vi "TestExec.Configure Setup and Dialog - Station.vi"(9 "Dialog":bool, 10 "SectAddFiles":string[](array[string])=["AdditionalConfig"] caption="Sections with Additional Files", 11 "Local Station Folder":path=path "C:/MTE/Test Executive/Config") -> (1 "Saved":bool, 2 "Data Out":variant, 3 "AppData out":refnum<class "Class.AppData.lvclass">)   [LabVIEW 2018]
uses:
  Common/Utils/TestExec/TestExec.WorkingDir.ctl
  <vilib>/KATE/Config/App Data/Class.AppData.lvclass
  Controls and Type Defs/TestExec.Config Dialog State.ctl
  <vilib>/Utility/config.llb/Write Key (String).vi
  <vilib>/KATE/Files/File Utils.lvlib
  <vilib>/Utility/config.llb/NI_LVConfig.lvlib
panel:
  out "Tab Control":enum32{"Inputs", "Data", "Outputs"}(tab)
  in  "Open Local Station File on Save":bool
  out "Exists_CfgFiles":bool[](array[boolean])
  out "Exists_ModeCfg":bool
  in  "Sequence":cluster{"Default":string}={"Default"="Undefined"}
  in  "Factory":cluster{"Location":string}={"Location"="Undefined"}
  in  "Route Check Enable":bool
  in  "Facility":cluster{"Name":string, "Location":string}={"Name"="Undefined", "Location"="Undefined"}
  in  "Station":T1={"Name"="Undefined", "PN"="Undefined", "SN"="Undefined", "Rev"="Undefined"}
  out "Additional Config Files":path[](array[path])
  in  "Mode Config File":path
  out "Local Station Config File":path=path "C:/MTE/Data/Eyetube Calibration/Capture"
  in  "Save":bool
  in  "Cancel":bool
  in  "Data Folders":T2[](array[typedef])=[{"Name"="ResultsLocalDir", "Path"=path "c:/MTE/Data/XML"}, {"Name"="ResultsExternalDir", "Path"=path "c:/MTE/Data/Results"}, {"Name"="DataArchiveDir", "Path"=path "c:/MTE/Data/Archive"}, {"Name"="DataSumArchiveDir", "Path"=path "c:/MTE/Data/ArchiveSum"}]
  # "Test Station Configuration"
  # "Name                                                                                                         Path"
  # "If this is empty, the default modes will be used."
  # "If a file is specified, it's contents will over write local settings."
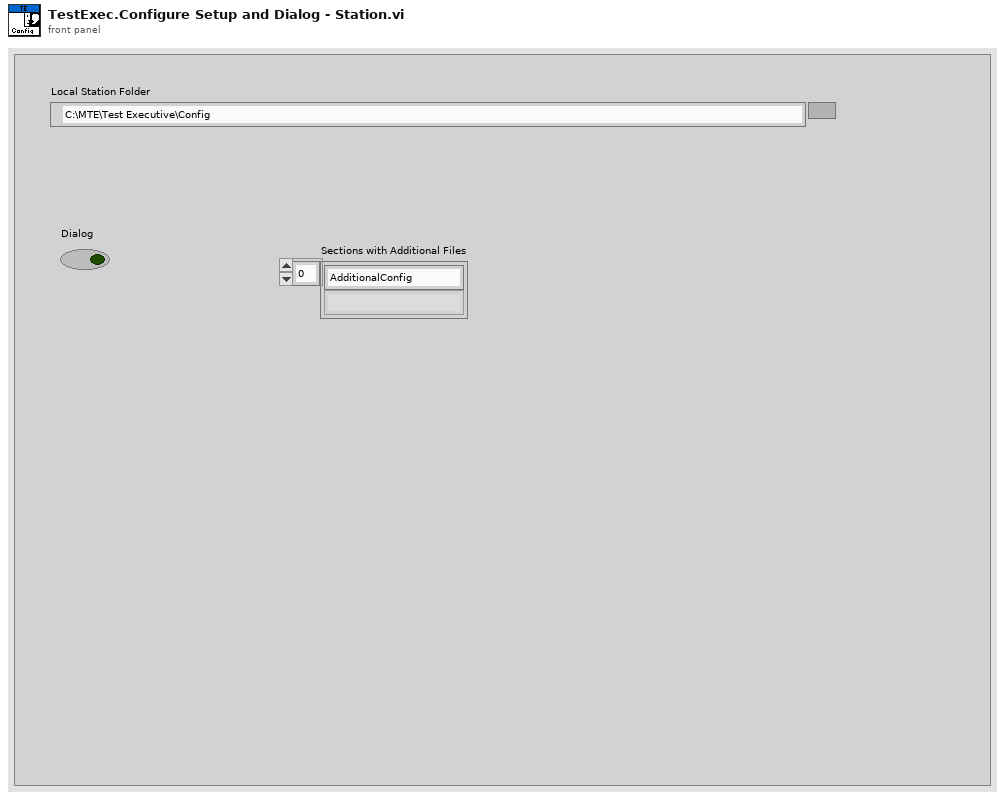
[diagram p1: front panel]
types:
  T1 = cluster{"Name":string, "PN":string, "SN":string, "Rev":string}
  T2 = typedef "TestExec.WorkingDir.ctl" = cluster{"Name":string, "Path":path}
  T3 = typedef "TestExec.Config Dialog State.ctl" = enum16{"Init", "Set Defaults", "Load Config", "Initialize Config", "Initialize Output", "Dialog", "Save", "Update Output", "Done"}
  T4 = enum32{"Invalid", "Standard", "Closed", "Hidden", "Minimized", "Maximized"}
  T5 = cluster{"Local Station Folder":path, "LocalCfgFile":path, "State":T3, "Save":bool, "Config":refnum<class "Class.AppData.lvclass">}
  T6 = typedef "NI_LVConfig.lvlib/Config Data RefNum.ctl" = refnum<k1>
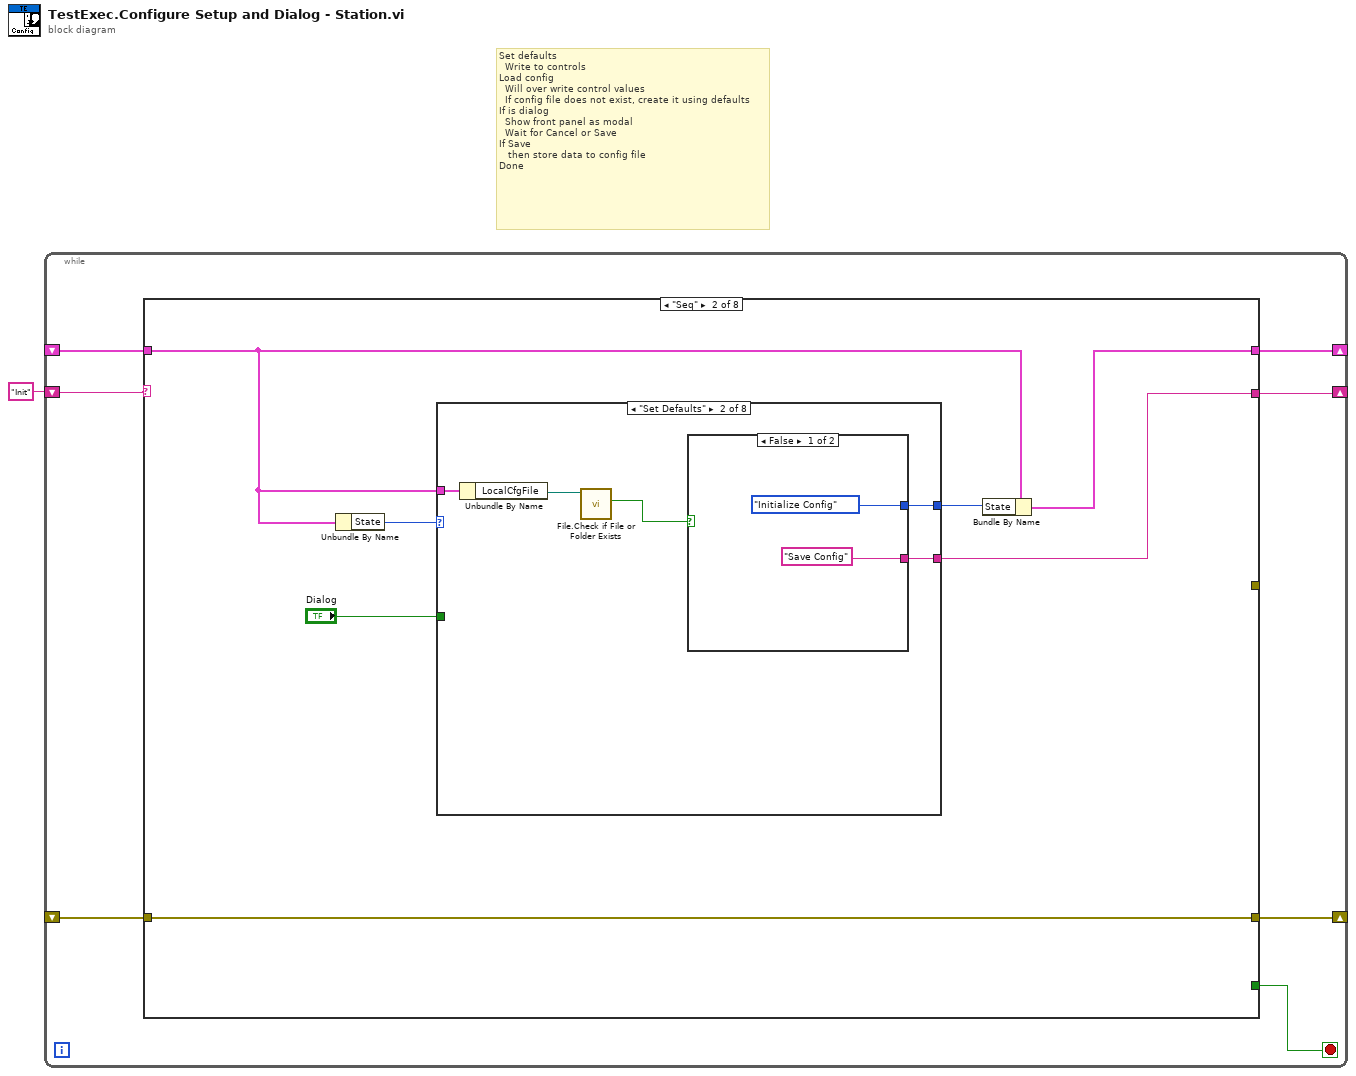
[diagram p0: block diagram]
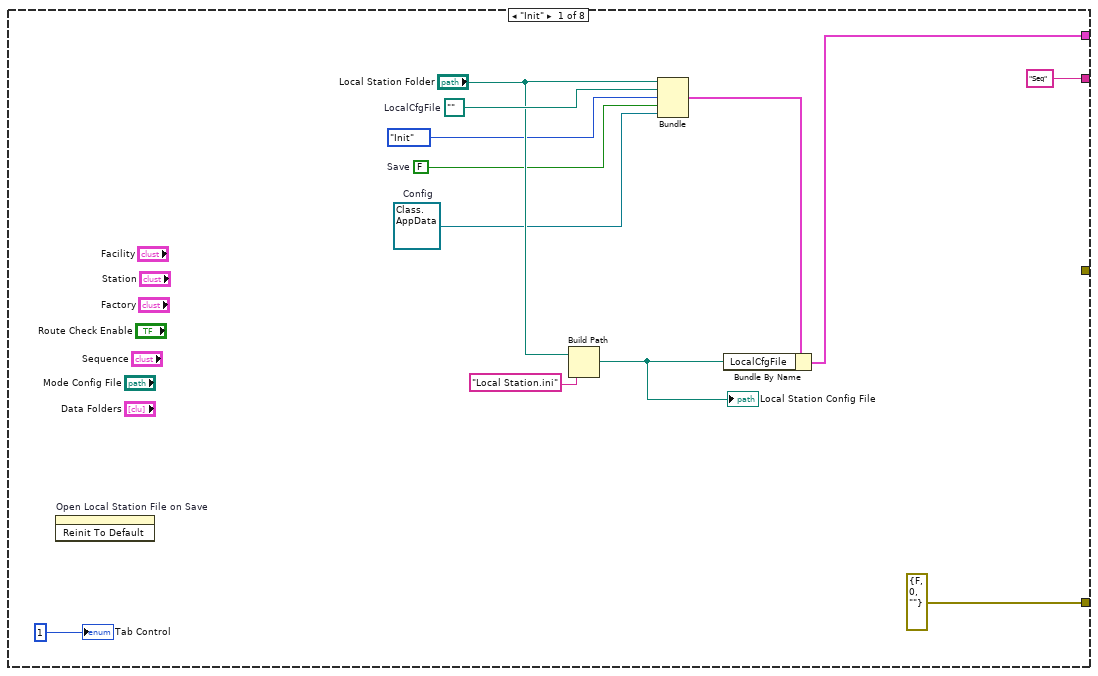
[diagram p2: hidden frame]
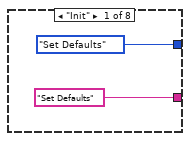
[diagram p3: hidden frame]
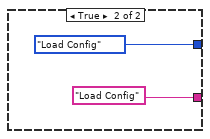
[diagram p4: hidden frame]
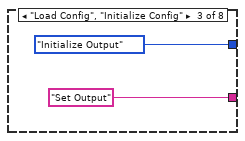
[diagram p5: hidden frame]
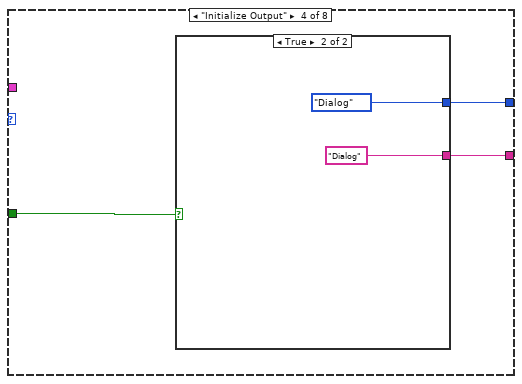
[diagram p6: hidden frame]
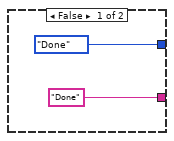
[diagram p7: hidden frame]
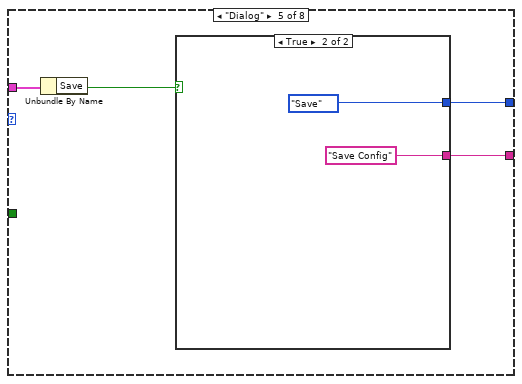
[diagram p8: hidden frame]
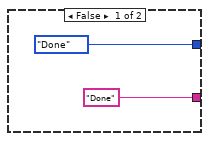
[diagram p9: hidden frame]
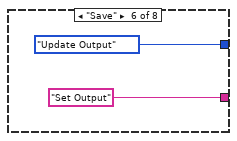
[diagram p10: hidden frame]
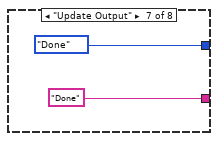
[diagram p11: hidden frame]
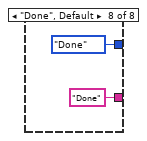
[diagram p12: hidden frame]
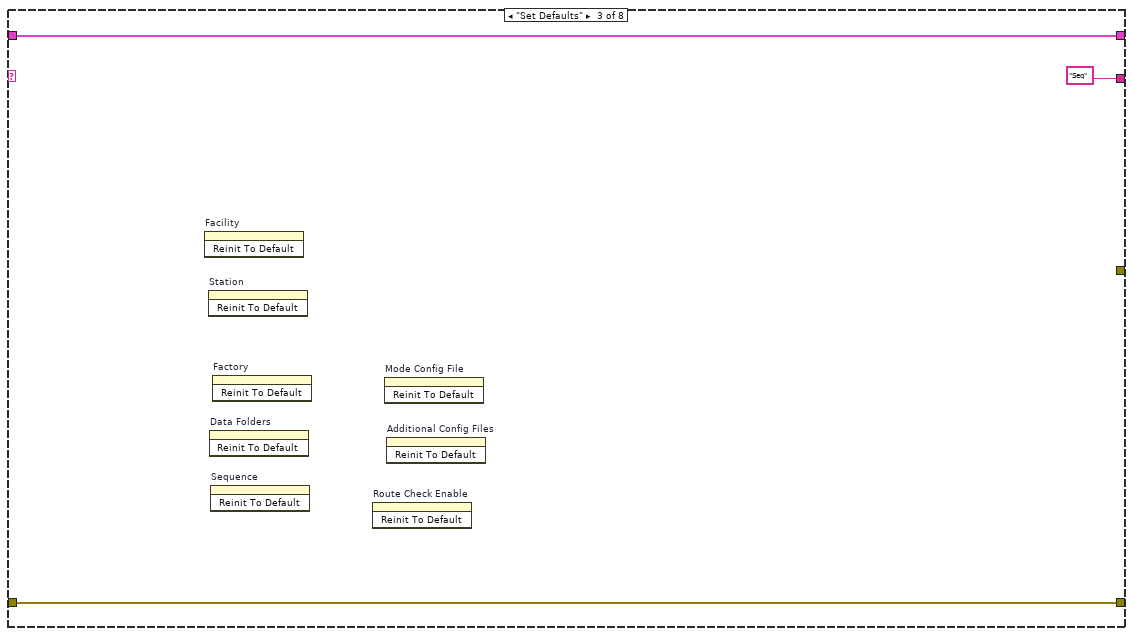
[diagram p13: hidden frame]
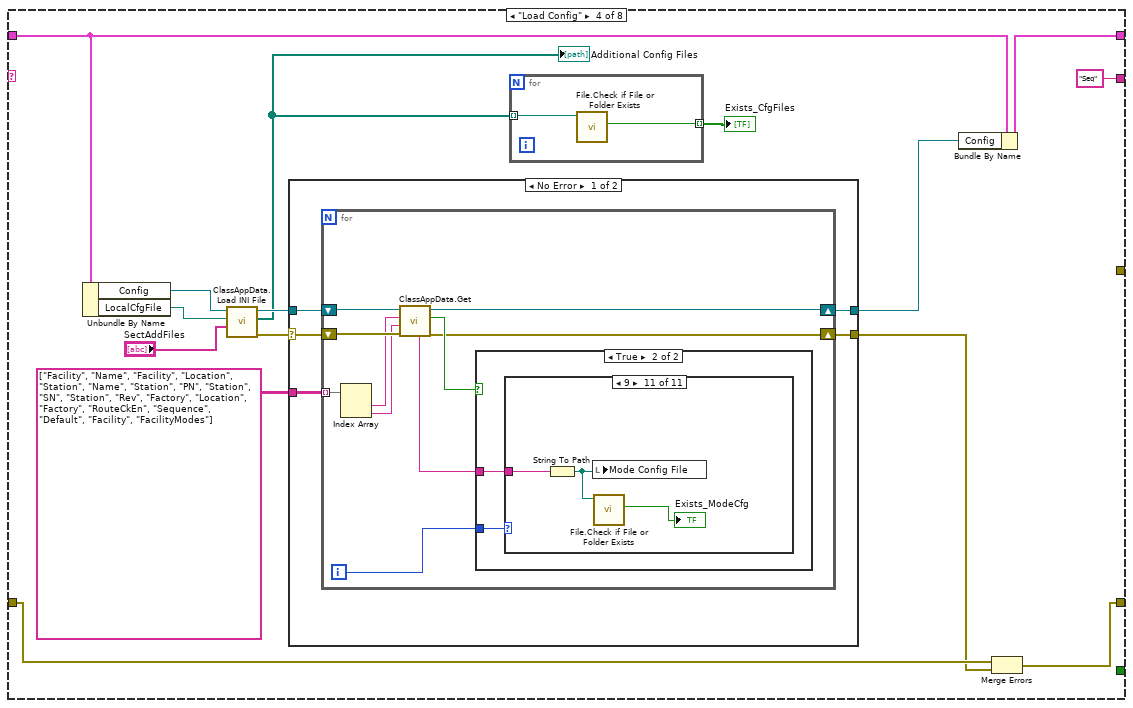
[diagram p14: hidden frame]
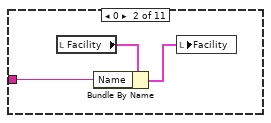
[diagram p17: hidden frame]
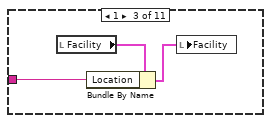
[diagram p18: hidden frame]
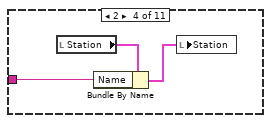
[diagram p19: hidden frame]
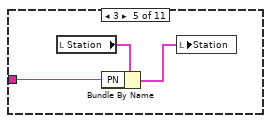
[diagram p20: hidden frame]
diagram:
  # "Set defaults\n  Write to controls\nLoad config\n  Will over write control values\n  If config file does not exist, create it using defaults\nIf is dialog\n  Show front panel as modal\n  Wait for Cancel or Save\nIf Save\n   then store data to config file\nDone"
  n1 = while {
    shift-right: [w6] -> _
    shift-left: _ -> [w8]
    shift-right: [w4] -> _
    shift-left: "Init" -> [w7]
    shift-right: [w2] -> _
    shift-left: _ -> [w3]
    stop <- w5 stop-if-true
    n2 = case shown="\"Seq\"" w7 {
      tunnel: w8 -> [_ w25 w63 w78 w150 w190 w200 w217]
      tunnel: [w15 w24 w63 w77 w149 w190 w199 w217] -> w6
      tunnel: ["Seq" w22 "Seq" "Seq" "Seq" "Seq" w198 "Done"] -> w4
      tunnel: [_ _ _ _ _ _ _ TRUE] -> w5
      tunnel: [_ _ _ _ w140 _ _ _] -> _
      tunnel: w3 -> [_ w21 w62 w68 w139 w196 w197 w218]
      tunnel: [errorcluster {"status"=FALSE, "code"=0, "source"=""} ("error constant") w21 w62 w66 w136 w196 w197 w218] -> w2
      frame "Init" {
        w10 = refnum<class "Class.AppData.lvclass"> refnum  # Config
        w13 = FALSE  # Save
        w18 = path ""  # LocalCfgFile
        n3 = invoke on="Open Local Station File on Save" class="Bool (strict)" method="Reinit To Default"() -> ()  [unwired: 3 in, 3 out]
        n4 = Build Path(base path="Local Station Folder", name or relative path="Local Station.ini") -> (appended path=w11:path)
        "Local Station Config File" <- w11
        n5 = Bundle("Local Station Folder"="Local Station Folder", "LocalCfgFile"=w18, "State"=TestExec.Config_Dialog_State."Init", "Save"=w13, "Config"=w10) -> (w16:T5)  [unwired: 1 in]
        n6 = Bundle By Name(cluster=w16, "LocalCfgFile"=w11) -> (w15:T5)
        "Tab Control" <- 1
      }
      frame "Seq" {
        n7 = Unbundle By Name(w25) -> ("State"=w27:T3)
        n8 = case shown="\"Set Defaults\"" w27 {
          tunnel: "Dialog" -> [_ _ _ w43 _ _ _ _]
          tunnel: w25 -> [_ w34 _ _ w49 _ _ _]
          tunnel: [TestExec.Config_Dialog_State."Set Defaults" ("State") w31 TestExec.Config_Dialog_State."Initialize Output" ("State") w42 w51 TestExec.Config_Dialog_State."Update Output" ("State") TestExec.Config_Dialog_State."Done" ("State") TestExec.Config_Dialog_State."Done" ("State")] -> w23
          tunnel: ["Set Defaults" w30 "Set Output" w41 w50 "Set Output" "Done" "Done"] -> w22
          frame "Init" {
          }
          frame "Set Defaults" {
            n9 = Unbundle By Name(w34) -> ("LocalCfgFile"=w33:path)
            n10 = call <vilib>:"File.Check if File or Folder Exists.vi"("Path"=w33) -> ("Exists"=w32:bool)  [unwired: 6 in, 4 out]
            n11 = case shown="False" w32 {
              tunnel: [TestExec.Config_Dialog_State."Initialize Config" ("State") TestExec.Config_Dialog_State."Load Config" ("State")] -> w31
              tunnel: ["Save Config" "Load Config"] -> w30
              frame False {
              }
              frame True {
              }
            }
          }
          frame "Load Config", "Initialize Config" {
          }
          frame "Initialize Output" {
            n12 = case shown="True" w43 {
              tunnel: [TestExec.Config_Dialog_State."Done" ("State") TestExec.Config_Dialog_State."Dialog" ("State")] -> w42
              tunnel: ["Done" "Dialog"] -> w41
              frame False {
              }
              frame True {
              }
            }
          }
          frame "Dialog" {
            n13 = Unbundle By Name(w49) -> ("Save"=w48:bool)
            n14 = case shown="True" w48 {
              tunnel: [TestExec.Config_Dialog_State."Done" ("State") TestExec.Config_Dialog_State."Save" ("State")] -> w51
              tunnel: ["Done" "Save Config"] -> w50
              frame False {
              }
              frame True {
              }
            }
          }
          frame "Save" {
          }
          frame "Update Output" {
          }
          frame "Done", Default {
          }
        }
        n15 = Bundle By Name(cluster=w25, "State"=w23) -> (w24:T5)
      }
      frame "Set Defaults" {
        n16 = invoke on="Facility" class="Clust (strict)" method="Reinit To Default"() -> ()  [unwired: 3 in, 3 out]
        n17 = invoke on="Station" class="Clust (strict)" method="Reinit To Default"() -> ()  [unwired: 3 in, 3 out]
        n18 = invoke on="Data Folders" class="Arr (strict)" method="Reinit To Default"() -> ()  [unwired: 3 in, 3 out]
        n19 = invoke on="Sequence" class="Clust (strict)" method="Reinit To Default"() -> ()  [unwired: 3 in, 3 out]
        n20 = invoke on="Factory" class="Clust (strict)" method="Reinit To Default"() -> ()  [unwired: 3 in, 3 out]
        n21 = invoke on="Route Check Enable" class="Bool (strict)" method="Reinit To Default"() -> ()  [unwired: 3 in, 3 out]
        n22 = invoke on="Mode Config File" class="Path" method="Reinit To Default"() -> ()  [unwired: 3 in, 3 out]
        n23 = invoke on="Additional Config Files" class="Arr (strict)" method="Reinit To Default"() -> ()  [unwired: 3 in, 3 out]
      }
      frame "Load Config" {
        n24 = Unbundle By Name(w78) -> ("Config"=w76:refnum<class "Class.AppData.lvclass">, "LocalCfgFile"=w75:path)
        n25 = call <vilib>:"ClassAppData.Load INI File.vi"("Sections that List RemoteFile"="SectAddFiles", "INI File"=w75, "Class - App Data in"=w76) -> ("error out"=w73:errorcluster, "Additional Cfg Files"=w69:path[], "Class - App Data out"=w74:refnum<class "Class.AppData.lvclass">)  [unwired: 6 in]
        "Additional Config Files" <- w69
        n26 = case shown="No Error" w73 {
          selector: w73 -> [w85 _]
          tunnel: w74 -> [w86 w133]
          tunnel: [w84 w133] -> w72
          tunnel: string[][] [["Facility", "Name"], ["Facility", "Location"], ["Station", "Name"], ["Station", "PN"], ["Station", "SN"], ["Station", "Rev"], ["Factory", "Location"], ["Factory", "RouteCkEn"], ["Sequence", "Default"], ["Facility", "FacilityModes"]] -> [w83 _]
          tunnel: [w82 _] -> w67
          frame No Error {
            n27 = for {
              shift-right: [w90] -> w84
              shift-left: w86 -> [w96]
              shift-right: [w89] -> w82
              shift-left: w85 -> [w95]
              tunnel: w83 -> [w94] mode=indexing
              i -> [w87]
              n28 = Index Array(array=w94) -> (element #1=w93:string, element #2=w92:string)  [unwired: 2 in]
              n29 = call <vilib>:"ClassAppData.Get.vi"("error in (no error)"=w95, "Name"=w92, "Section"=w93, "Class - App Data in"=w96) -> ("error out"=w89:errorcluster, "Found"=w91:bool, "Class - App Data out"=w90:refnum<class "Class.AppData.lvclass">, "String Data"=w88:string)  [unwired: 3 in, 1 out]
              n30 = case shown="True" w91 {
                tunnel: w88 -> [_ w97]
                tunnel: w87 -> [_ w98]
                frame False {
                  # "Skip"
                }
                frame True {
                  n31 = case shown="9" w98 {
                    tunnel: w97 -> [_ w99 w102 w105 w108 w111 w114 w117 w125 w127 w132]
                    frame Default {
                    }
                    frame 0 {
                      n32 = local read "Facility"() -> (w101:cluster{"Name":string, "Location":string})
                      n33 = Bundle By Name(cluster=w101, "Name"=w99) -> (w100:cluster{"Name":string, "Location":string})
                      n34 = local write "Facility"(w100) -> ()
                    }
                    frame 1 {
                      n35 = local read "Facility"() -> (w104:cluster{"Name":string, "Location":string})
                      n36 = Bundle By Name(cluster=w104, "Location"=w102) -> (w103:cluster{"Name":string, "Location":string})
                      n37 = local write "Facility"(w103) -> ()
                    }
                    frame 2 {
                      n38 = local read "Station"() -> (w107:T1)
                      n39 = Bundle By Name(cluster=w107, "Name"=w105) -> (w106:T1)
                      n40 = local write "Station"(w106) -> ()
                    }
                    frame 3 {
                      n41 = local read "Station"() -> (w110:T1)
                      n42 = Bundle By Name(cluster=w110, "PN"=w108) -> (w109:T1)
                      n43 = local write "Station"(w109) -> ()
                    }
                    frame 4 {
                      n44 = local read "Station"() -> (w113:T1)
                      n45 = Bundle By Name(cluster=w113, "SN"=w111) -> (w112:T1)
                      n46 = local write "Station"(w112) -> ()
                    }
                    frame 5 {
                      n47 = local read "Station"() -> (w116:T1)
                      n48 = Bundle By Name(cluster=w116, "Rev"=w114) -> (w115:T1)
                      n49 = local write "Station"(w115) -> ()
                    }
                    frame 6 {
                      n50 = local read "Factory"() -> (w119:cluster{"Location":string})
                      n51 = Bundle By Name(cluster=w119, "Location"=w117) -> (w118:cluster{"Location":string})
                      n52 = local write "Factory"(w118) -> ()
                    }
                    frame 7 {
                      n53 = To Upper Case(1:w125) -> (0:w126:string)
                      n54 = Equal?(x="1" ("y"), y=w125) -> (x = y?=w121:bool)
                      n55 = Equal?(x=w126, y="TRUE") -> (x = y?=w122:bool)
                      n56 = Or(x=w121, y=w122) -> (x .or. y?=w120:bool)
                      n57 = local write "Route Check Enable"(w120) -> ()
                    }
                    frame 8 {
                      n58 = local read "Sequence"() -> (w129:cluster{"Default":string})
                      n59 = Bundle By Name(cluster=w129, "Default"=w127) -> (w128:cluster{"Default":string})
                      n60 = local write "Sequence"(w128) -> ()
                    }
                    frame 9 {
                      n61 = String To Path(string=w132) -> (path=w131:path)
                      n62 = local write "Mode Config File"(w131) -> ()
                      n63 = call <vilib>:"File.Check if File or Folder Exists.vi"("Path"=w131) -> ("Exists"=→"Exists_ModeCfg":bool)  [unwired: 6 in, 4 out]
                    }
                  }
                }
              }
            }
          }
          frame Error {
          }
        }
        n64 = for {
          tunnel: w69 -> [w81] mode=indexing
          tunnel: [w80] -> w70 mode=indexing
          n65 = call <vilib>:"File.Check if File or Folder Exists.vi"("Path"=w81) -> ("Exists"=w80:bool)  [unwired: 6 in, 4 out]
        }
        "Exists_CfgFiles" <- w70
        n66 = Bundle By Name(cluster=w78, "Config"=w72) -> (w77:T5)
        n67 = Merge Errors(w68, w67) -> (w66:errorcluster)
      }
      frame "Save Config" {
        n68 = Unbundle By Name(w150) -> ("LocalCfgFile"=w144:path, "Config"=w146:refnum<class "Class.AppData.lvclass">)
        n69 = call <vilib>:"Open Config Data.vi"("create file if necessary (T)"=TRUE, "configuration file path"=w144) -> ("error out"=w135:errorcluster, "refnum"=w143:T6)  [unwired: 7 in, 1 out]
        n70 = for {
          shift-right: [w162] -> w148
          shift-left: w146 -> [w165]
          shift-right: [w161] -> w138
          shift-left: errorcluster {"status"=FALSE, "code"=0, "source"=""} ("error constant") -> [w164]
          tunnel: string[][] [["Facility", "Name"], ["Facility", "Location"], ["Station", "Name"], ["Station", "PN"], ["Station", "SN"], ["Station", "Rev"], ["Factory", "Location"], ["Factory", "RouteCkEn"], ["Sequence", "Default"], ["Facility", "FacilityModes"]] -> [w163] mode=indexing
          shift-right: [w152] -> w137
          shift-left: w135 -> [w157]
          shift-right: [w153] -> w141
          shift-left: w143 -> [w158]
          i -> [w160]
          n71 = Index Array(array=w163) -> (element #1=w155:string, element #2=w156:string)  [unwired: 2 in]
          n72 = case shown="9" w160 {
            tunnel: [_ w166 w168 w171 w173 w175 w177 w179 w180 w184 w187] -> w154
            frame Default {
            }
            frame 0 {
              n73 = local read "Facility"() -> (w167:cluster{"Name":string, "Location":string})
              n74 = Unbundle By Name(w167) -> ("Name"=w166:string)
            }
            frame 1 {
              n75 = local read "Facility"() -> (w169:cluster{"Name":string, "Location":string})
              n76 = Unbundle By Name(w169) -> ("Location"=w168:string)
            }
            frame 2 {
              n77 = local read "Station"() -> (w170:T1)
              n78 = Unbundle By Name(w170) -> ("Name"=w171:string)
            }
            frame 3 {
              n79 = local read "Station"() -> (w172:T1)
              n80 = Unbundle By Name(w172) -> ("PN"=w173:string)
            }
            frame 4 {
              n81 = local read "Station"() -> (w174:T1)
              n82 = Unbundle By Name(w174) -> ("SN"=w175:string)
            }
            frame 5 {
              n83 = local read "Station"() -> (w176:T1)
              n84 = Unbundle By Name(w176) -> ("Rev"=w177:string)
            }
            frame 6 {
              n85 = local read "Factory"() -> (w178:cluster{"Location":string})
              n86 = Unbundle By Name(w178) -> ("Location"=w179:string)
            }
            frame 7 {
              n87 = local read "Route Check Enable"() -> (w181:bool)
              n88 = Select(t="TRUE" ("y"), s=w181, f="FALSE" ("y")) -> (s? t:f=w180:string)
            }
            frame 8 {
              n89 = local read "Sequence"() -> (w185:cluster{"Default":string})
              n90 = Unbundle By Name(w185) -> ("Default"=w184:string)
            }
            frame 9 {
              n91 = local read "Mode Config File"() -> (w188:path)
              n92 = call <vilib>:"File.Check if File or Folder Exists.vi"("Path"=w188) -> ("Exists"=w189:bool, "Dup Path"=w186:path)  [unwired: 6 in, 3 out]
              n93 = Path To String(path=w186) -> (string=w187:string)
              n94 = local write "Exists_ModeCfg"(w189) -> ()
            }
          }
          n95 = To Variant(anything=w154) -> (Variant=w159:variant)
          n96 = call <vilib>:"ClassAppData.Set.vi"("Section"=w155, "error in (no error)"=w164, "Value"=w159, "Name"=w156, "Class - App Data in"=w165) -> ("error out"=w161:errorcluster, "Class - App Data out"=w162:refnum<class "Class.AppData.lvclass">)  [unwired: 4 in, 1 out]
          n97 = call-poly <vilib>:"Write Key.vi"("section"=w155, "error in (no error)"=w157, "value"=w154, "key"=w156, "refnum"=w158) -> ("error out"=w152:errorcluster, "refnum out"=w153:T6)  [unwired: 4 in, 1 out]
        }
        n98 = call <vilib>:"Close Config Data.vi"("error in (no error)"=w137, "write file if changed (T)"=TRUE, "refnum"=w141) -> ("error out"=w140:errorcluster)  [unwired: 7 in, 1 out]
        n99 = Bundle By Name(cluster=w150, "Config"=w148) -> (w149:T5)
        n100 = Merge Errors(w139, w138, w137) -> (w136:errorcluster)
      }
      frame "Set Output" {
        n101 = Unbundle By Name(w190) -> ("Save"=→"Saved":bool, "Config"=w192:refnum<class "Class.AppData.lvclass">)
        n102 = call <vilib>:"ClassAppData.Get All.vi"("Class - App Data in"=w192) -> ("Data Out"=→"Data Out":variant, "Class - App Data out"=→"AppData out":refnum<class "Class.AppData.lvclass">)  [unwired: 8 in, 1 out]
      }
      frame "Dialog" {
        n103 = control-ref of="This VI"() -> (w206:refnum<vi>)
        n104 = invoke class="VI" method="FP.Open"(reference=w206, "Activate"=TRUE ("Activate?"), "State"=T4."Standard") -> (reference out=w203:refnum<vi>, error out=w202:errorcluster)  [unwired: 2 in, 3 out]
        n105 = Close Reference(reference=w203, error in (no error)=w202) -> (error out=w201:errorcluster)
        n106 = while {
          tunnel: w201 -> [_]
          shift-right: [w208] -> w199
          shift-left: w200 -> [w209]
          tunnel: [w207] -> w198
          stop <- w210 stop-if-true
          n107 = event shown="[0] \"Cancel\", \"Save\": Value Change;  Panel Close" {
            selector: _ -> [_]
            dyn-events: _ -> [_]
            timeout: _ -> [_]
            tunnel: [TRUE] -> w210
            tunnel: w209 -> [w213]
            tunnel: [w212] -> w208
            tunnel: ["Seq"] -> w207
            event "Cancel", "Save": Value Change; Panel Close {
              n108 = event-data() -> ()  [unwired: 1 in, 3 out]
              n109 = Bundle By Name(cluster=w213, "Save"="Save") -> (w212:T5)
            }
          }
        }
      }
      frame "Done", Default {
        w220 = TRUE  # Normal(T)/Debug(F)
        n110 = local read "Dialog"() -> (w221:bool)
        n111 = And(x=w221, y=w220) -> (x .and. y?=w219:bool)
        n112 = case shown="True" "Open Local Station File on Save" {
          tunnel: w217 -> [_ w226]
          frame False {
          }
          frame True {
            n113 = Unbundle By Name(w226) -> ("LocalCfgFile"=w225:path)
            n114 = call <vilib>:"File.Open File or Folder.vi"("Path"=w225) -> ("Error Out"=w224:errorcluster)  [unwired: 10 in]
            n115 = call <vilib>:"Clear Errors.vi"("error in (no error)"=w224) -> ()  [unwired: 5 in, 2 out]
          }
        }
        n116 = case shown="True" w219 {
          tunnel: [_ w227] -> _
          frame False {
          }
          frame True {
            n117 = control-ref of="This VI"() -> (w230:refnum<vi>)
            n118 = invoke class="VI" method="FP.Close"(reference=w230) -> (reference out=w229:refnum<vi>, error out=w228:errorcluster)  [unwired: 2 in, 1 out]
            n119 = Close Reference(reference=w229, error in (no error)=w228) -> (error out=w227:errorcluster)
          }
        }
      }
    }
  }
